vi "asyncvistopsfromlast.vi"(10 "subchannel":i32, 11 "channel":T1) -> (3 "other channel out":T1)   [LabVIEW 2020, in "Tests Event MessengerM.lvclass"]
uses:
  Tests Event MessengerM.lvclass
  Tests Event MessengerM.lvclass/Tests Event MessengerM.ctl
  source/Event MessengerM.lvlib
  source/))Channel.ctl
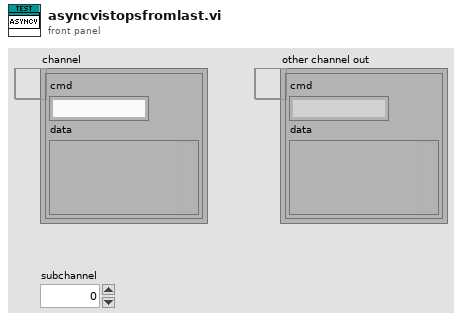
[diagram p1: front panel]
types:
  T1 = typedef "Event MessengerM.lvlib/))Channel.ctl" = refnum<queue>
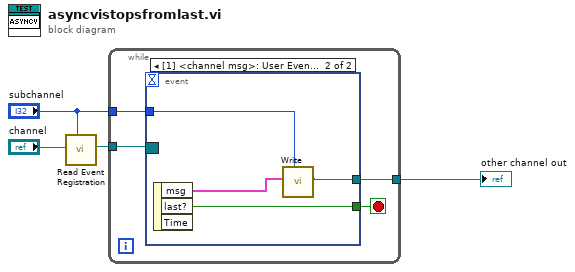
[diagram p0: block diagram]
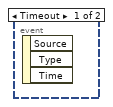
[diagram p2: hidden frame]
diagram:
  n1 = call "Read Event Registration.vi"("subchannel"="subchannel", "channel"="channel") -> ("event registration refnum"=w3:refnum<event-registration>)  [unwired: 9 in]
  n2 = while {
    tunnel: w3 -> [w8]
    tunnel: [w6] -> w2
    tunnel: "subchannel" -> [w5]
    stop <- w7 stop-if-true
    n3 = event shown="[1] <channel msg>: User Event" {
      selector: w8 -> [_ _]
      dyn-events: _ -> [_ _]
      timeout: _ -> [_ _]
      tunnel: [_ w12] -> w7
      tunnel: [_ w10] -> w6
      tunnel: w5 -> [_ w9]
      event Timeout {
        n4 = event-data() -> ()  [unwired: 1 in, 3 out]
      }
      event User Event {
        n5 = event-data() -> ("msg"=w11:cluster{"cmd":string, "data":variant}, "last?"=w12:bool)  [unwired: 1 in, 1 out]
        n6 = call "Write.vi"("subchannel (0)"=w9, "element"=w11) -> ("channel"=w10:T1)  [unwired: 8 in, 1 out]
      }
    }
  }
  "other channel out" <- w2
